vi "MaxiGauge EPICS2.vi"() -> ()   [LabVIEW 2015]
uses:
  <vilib>/Platform/TimedLoop/XDataNode/timing_clust.ctl
  <vilib>/Platform/TimedLoop/XDataNode/nitl_modes.ctl
  <vilib>/Platform/TimedLoop/XDataNode/wakeup.ctl
  <userlib>/caLab/Private/Get_PV-1D.vi
  <userlib>/caLab/Private/Put_DBL-1D_PV-1D.vi
  <vilib>/platform/TimedLoop/XDataNode/XDataNode.xnode
  <vilib>/Platform/TimedLoop/XDataNode/XDNodeRunTimeDep.lvlib
panel:
  out "Relay E":string
  out "Error out":errorcluster
  out "Maxigauge COMPORT":string
  out "APX:SEN6_STS":bool
  out "APX:SEN5_STS":bool
  out "APX:SEN4_STS":bool
  out "APX:SEN3_STS":bool
  out "APX:SEN2_STS":bool
  out "APX:SEN1_STS":bool
  out "APX:SEN6_VAL":dbl
  out "APX:SEN5_VAL":dbl
  out "APX:SEN4_VAL":dbl format="%#_3g"
  out "APX:SEN3_VAL":dbl format="%#_3g"
  out "APX:SEN2_VAL":dbl format="%#_3g"
  out "APX:SEN1_VAL":dbl
  out "APX:SEN6_OFF":bool
  out "APX:SEN6_ON":bool
  out "APX:SEN5_OFF":bool
  out "APX:SEN5_ON":bool
  out "APX:SEN4_OFF":bool
  out "APX:SEN4_ON":bool
  out "APX:SEN3_OFF":bool
  out "APX:SEN3_ON":bool
  out "APX:SEN2_OFF":bool
  out "APX:SEN2_ON":bool
  out "APX:SEN1_OFF":bool
  out "APX:SEN1_ON":bool
  out "APX:SP_SES100":bool
  out "MaxiGauge":dbl[](array[numeric])
  out "P torr":dbl[](array[numeric])
  in  "STOP":bool
  # "Ch 1\nGMP\nCh 6\nGMP\nCh 2\nGCC\nCh 4\nGHC\nCh 5\nGHC\n\nGMP"
  # "Send measured values to EPICS [COM8]"
  # "Relay E"
  # "K"
  # "EPICS PV name"
  # "N"
  # "APX:HPC100"
  # "APX:HPC100"
  # "APX:HPC01"
  # "APX:HPC"
  # "APX:HPC"
  # "N"
  # "APX:AP1"
  # "APX:PREP"
  # "APX:AP2"
  # "APX:Tsample"
  # "APX:AP1"
  # "APX:Tpiezo"
  # "APX:Thpc"
  # "APX:AP2"
  # "APX:PREP"
  # "APX:HPC01"
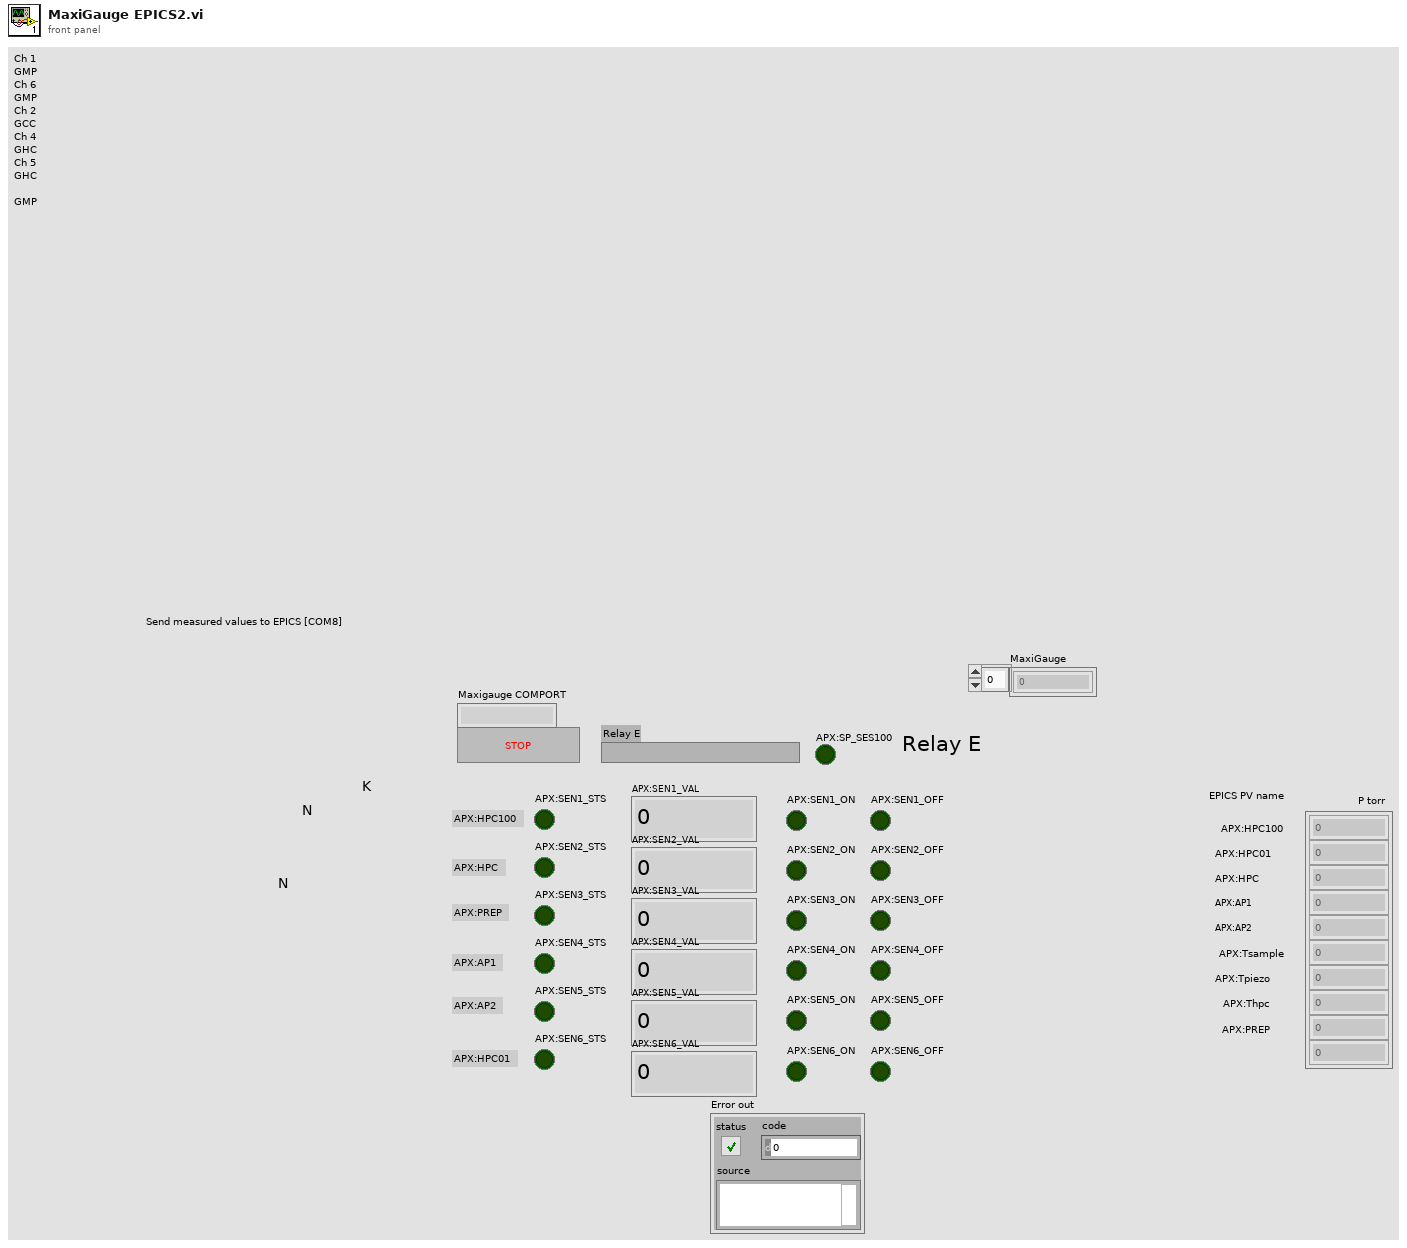
[diagram p1: front panel]
types:
  T1 = typedef "XDNodeRunTimeDep.lvlib/timing_clust.ctl" = cluster{"Expected End [f-1]":u64, "Actual End [f-1]":u64, "Finished Late? [f-1]":bool, "Expected End [i-1]":u64, "Actual End [i-1]":u64, "Finished Late? [i-1]":bool, "Expected Start [i]":u64, "Actual Start [i]":u64, "Expected Start [f]":u64, "Actual Start [f]":u64, "Source Name":string, "Structure Name":string, "Period":i64, "Deadline":i64, "Offset":i64, "Start":i64, "Priority":i32, "Timeout":i32, "Mode":T2, "Wakeup Reason":T3, "Error":errorcluster, "Source Type":string, "Secondary Source Type":string, "Global End Time":u64, "Global Start Time":u64, "Frame Duration":u64, "Iteration Duration":u64, "Assigned CPU":i32, "I/O Scan Engine Mode":u32}
  T2 = typedef "XDNodeRunTimeDep.lvlib/nitl_modes.ctl" = enum32{"No Change", "Process missed periods, maintain original phase", "Discard missed periods, maintain original phase", "Process missed periods, ignore original phase", "Discard missed periods, ignore original phase"}
  T3 = typedef "XDNodeRunTimeDep.lvlib/wakeup.ctl" = enum32{"Normal", "Aborted", "Asynchronous wakeup", "Timing source error", "Timed loop error", "Timeout"}
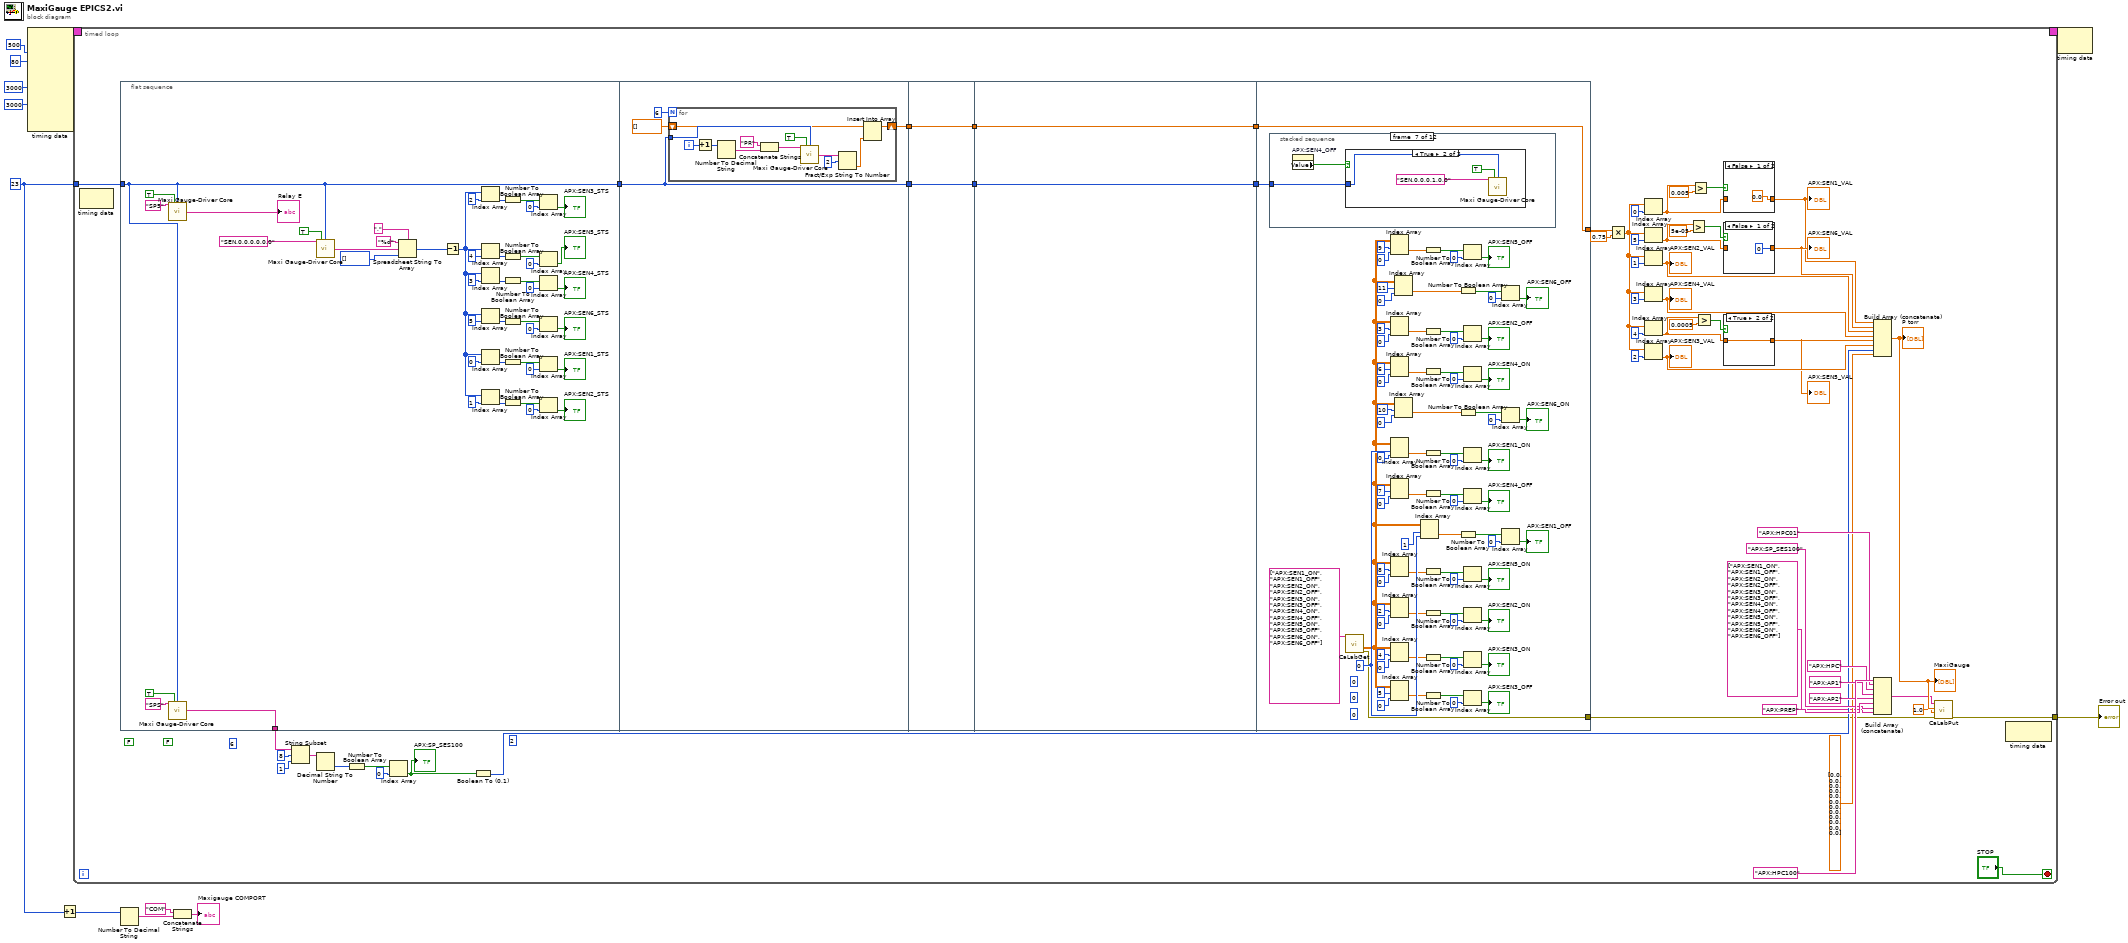
[diagram p0: block diagram]
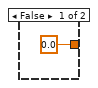
[diagram p2: hidden frame]
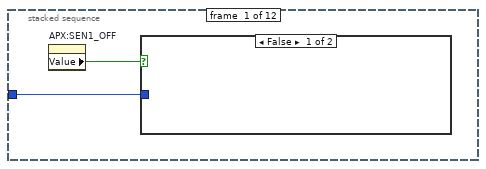
[diagram p3: hidden frame]
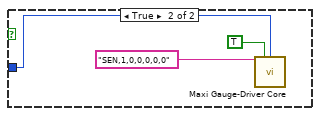
[diagram p4: hidden frame]
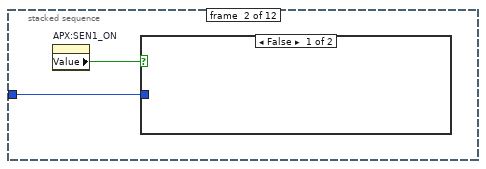
[diagram p5: hidden frame]
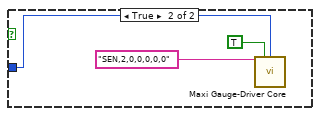
[diagram p6: hidden frame]
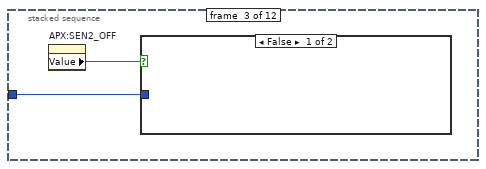
[diagram p7: hidden frame]
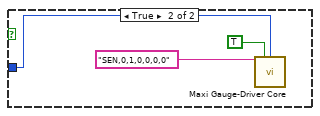
[diagram p8: hidden frame]
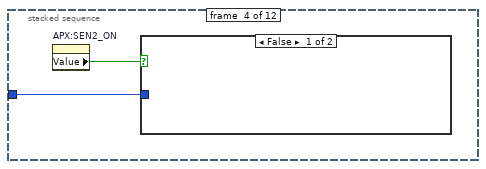
[diagram p9: hidden frame]
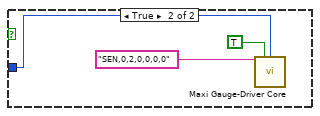
[diagram p10: hidden frame]
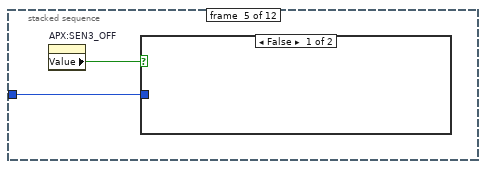
[diagram p11: hidden frame]
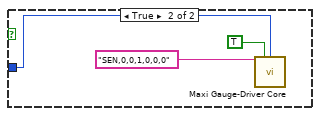
[diagram p12: hidden frame]
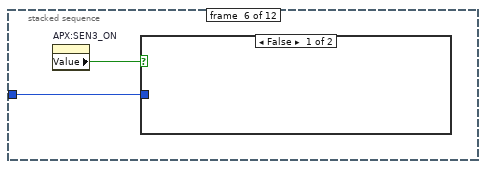
[diagram p13: hidden frame]
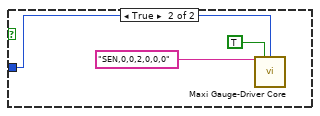
[diagram p14: hidden frame]
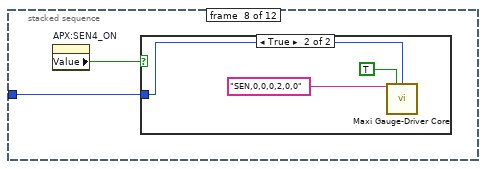
[diagram p16: hidden frame]
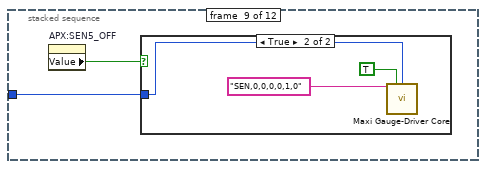
[diagram p18: hidden frame]
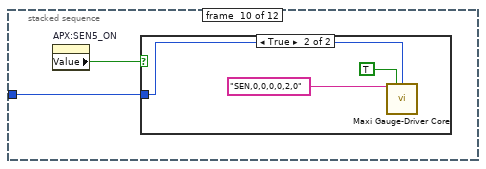
[diagram p20: hidden frame]
diagram:
  w8 = 23 ("Port")
  n1 = node-c288(i64 500 ("Period"), 80 ("Priority"), i64 3000 ("Deadline"), 3000 ("Timeout")) -> (w12:T1)  [unwired: 6 in]
  n2 = Increment(x=w8) -> (x+1=w7:i32)
  n3 = timed-loop {
    tunnel: w8 -> [w46]
    timing: w12 -> [_]
    timing-out: [_] -> w11
    tunnel: [w17] -> w3
    stop <- "STOP" stop-if-true
    (unwired) FALSE ("SES-100HVoff")
    (unwired) FALSE ("SES-100HVon")
    (unwired) 6
    (unwired) 2 ("index")
    n4 = node-c288() -> ()  [unwired: 1 in, 1 out]
    n5 = flat-sequence {
      tunnel: w46 -> [w73]
      tunnel: [w73] -> w45
      tunnel: [w113] -> w42
      tunnel: w45 -> [w116]
      tunnel: [w117] -> w22
      tunnel: [w116] -> w21
      tunnel: w22 -> [w133]
      tunnel: [w133] -> w16
      tunnel: w21 -> [w132]
      tunnel: [w132] -> w14
      tunnel: w16 -> [w135]
      tunnel: [w135] -> w15
      tunnel: w14 -> [w134]
      tunnel: [w134] -> w13
      tunnel: [w211] -> w58
      tunnel: w15 -> [w211]
      tunnel: w13 -> [w209]
      tunnel: [w136] -> w18
      frame #0 {
        n6 = call "Maxi Gauge-Driver Core.vi"("Command"="SP5", "Write/Read"=TRUE, "Port"=w73) -> ("String Out"=→"Relay E":string)  [unwired: 3 in, 9 out]
        n7 = call "Maxi Gauge-Driver Core.vi"("Command"="SPS", "Write/Read"=TRUE, "Port"=w73) -> ("String Out"=w113:string)  [unwired: 3 in, 9 out]
        n8 = call "Maxi Gauge-Driver Core.vi"("Command"="SEN,0,0,0,0,0,0", "Write/Read"=TRUE, "Port"=w73) -> ("String Out"=w109:string)  [unwired: 3 in, 9 out]
        n9 = Spreadsheet String To Array(delimiter (Tab)=",", format string="%d", spreadsheet string=w109, array type (2D Dbl)=i16[] []) -> (array=w105:i16[])
        n10 = Decrement(x=w105) -> (x-1=w80:i16[])
        n11 = Index Array(array=w80, index=2) -> (element=w95:i16)
        n12 = Index Array(array=w80, index=4) -> (element=w87:i16)
        n13 = Index Array(array=w80, index=3) -> (element=w91:i16)
        n14 = Index Array(array=w80, index=5) -> (element=w83:i16)
        n15 = Index Array(array=w80, index=0) -> (element=w104:i16)
        n16 = Index Array(array=w80, index=1) -> (element=w99:i16)
        n17 = Number To Boolean Array(number=w95) -> (Boolean array=w94:bool[])
        n18 = Number To Boolean Array(number=w87) -> (Boolean array=w86:bool[])
        n19 = Number To Boolean Array(number=w91) -> (Boolean array=w90:bool[])
        n20 = Number To Boolean Array(number=w83) -> (Boolean array=w82:bool[])
        n21 = Number To Boolean Array(number=w104) -> (Boolean array=w103:bool[])
        n22 = Number To Boolean Array(number=w99) -> (Boolean array=w98:bool[])
        n23 = Index Array(array=w94, index=0) -> (element=→"APX:SEN3_STS":bool)
        n24 = Index Array(array=w86, index=0) -> (element=→"APX:SEN5_STS":bool)
        n25 = Index Array(array=w90, index=0) -> (element=→"APX:SEN4_STS":bool)
        n26 = Index Array(array=w82, index=0) -> (element=→"APX:SEN6_STS":bool)
        n27 = Index Array(array=w103, index=0) -> (element=→"APX:SEN1_STS":bool)
        n28 = Index Array(array=w98, index=0) -> (element=→"APX:SEN2_STS":bool)
      }
      frame #1 {
        n29 = for {
          N: 6 -> [_]
          tunnel: w116 -> [w123]
          shift-right: [w120] -> w117
          shift-left: dbl[] [] -> [w121]
          i -> [w125]
          n30 = Increment(x=w125) -> (x+1=w128:i32)
          n31 = Number To Decimal String(number=w128) -> (decimal integer string=w131:string)  [unwired: 1 out]
          n32 = Concatenate Strings("PR", w131) -> (w129:string)
          n33 = call "Maxi Gauge-Driver Core.vi"("Command"=w129, "Write/Read"=TRUE, "Port"=w123) -> ("String Out"=w127:string)  [unwired: 3 in, 9 out]
          n34 = Fract/Exp String To Number(string=w127, offset=2 ("offset (0)")) -> (number=w122:dbl)  [unwired: 3 out]
          n35 = Insert Into Array(array=w121, new element=w122) -> (w120:dbl[])  [unwired: 1 in]
        }
      }
      frame #2 {
      }
      frame #3 {
      }
      frame #4 {
        (unwired) 0 ("index (col)")
        w199 = 0 ("index")
        (unwired) 0 ("disabled index (col)")
        (unwired) 0 ("index (row)")
        n36 = stacked-sequence {
          tunnel: w209 -> [w212 w217 w222 w227 w232 w237 w242 w247 w252 w257 w262 w267]
          frame #0 {
            n37 = property on="APX:SEN1_OFF" class="Bool (strict)"() -> ("Value"=w213:bool)  [unwired: 2 in, 2 out]
            n38 = case shown="False" w213 {
              tunnel: w212 -> [_ w214]
              frame False {
              }
              frame True {
                n39 = call "Maxi Gauge-Driver Core.vi"("Command"="SEN,1,0,0,0,0,0", "Write/Read"=TRUE, "Port"=w214) -> ()  [unwired: 3 in, 10 out]
              }
            }
          }
          frame #1 {
            n40 = property on="APX:SEN1_ON" class="Bool (strict)"() -> ("Value"=w218:bool)  [unwired: 2 in, 2 out]
            n41 = case shown="False" w218 {
              tunnel: w217 -> [_ w219]
              frame False {
              }
              frame True {
                n42 = call "Maxi Gauge-Driver Core.vi"("Command"="SEN,2,0,0,0,0,0", "Write/Read"=TRUE, "Port"=w219) -> ()  [unwired: 3 in, 10 out]
              }
            }
          }
          frame #2 {
            n43 = property on="APX:SEN2_OFF" class="Bool (strict)"() -> ("Value"=w223:bool)  [unwired: 2 in, 2 out]
            n44 = case shown="False" w223 {
              tunnel: w222 -> [_ w225]
              frame False {
              }
              frame True {
                n45 = call "Maxi Gauge-Driver Core.vi"("Command"="SEN,0,1,0,0,0,0", "Write/Read"=TRUE, "Port"=w225) -> ()  [unwired: 3 in, 10 out]
              }
            }
          }
          frame #3 {
            n46 = property on="APX:SEN2_ON" class="Bool (strict)"() -> ("Value"=w228:bool)  [unwired: 2 in, 2 out]
            n47 = case shown="False" w228 {
              tunnel: w227 -> [_ w230]
              frame False {
              }
              frame True {
                n48 = call "Maxi Gauge-Driver Core.vi"("Command"="SEN,0,2,0,0,0,0", "Write/Read"=TRUE, "Port"=w230) -> ()  [unwired: 3 in, 10 out]
              }
            }
          }
          frame #4 {
            n49 = property on="APX:SEN3_OFF" class="Bool (strict)"() -> ("Value"=w233:bool)  [unwired: 2 in, 2 out]
            n50 = case shown="False" w233 {
              tunnel: w232 -> [_ w234]
              frame False {
              }
              frame True {
                n51 = call "Maxi Gauge-Driver Core.vi"("Command"="SEN,0,0,1,0,0,0", "Write/Read"=TRUE, "Port"=w234) -> ()  [unwired: 3 in, 10 out]
              }
            }
          }
          frame #5 {
            n52 = property on="APX:SEN3_ON" class="Bool (strict)"() -> ("Value"=w238:bool)  [unwired: 2 in, 2 out]
            n53 = case shown="False" w238 {
              tunnel: w237 -> [_ w240]
              frame False {
              }
              frame True {
                n54 = call "Maxi Gauge-Driver Core.vi"("Command"="SEN,0,0,2,0,0,0", "Write/Read"=TRUE, "Port"=w240) -> ()  [unwired: 3 in, 10 out]
              }
            }
          }
          frame #6 {
            n55 = property on="APX:SEN4_OFF" class="Bool (strict)"() -> ("Value"=w243:bool)  [unwired: 2 in, 2 out]
            n56 = case shown="True" w243 {
              tunnel: w242 -> [_ w245]
              frame False {
              }
              frame True {
                n57 = call "Maxi Gauge-Driver Core.vi"("Command"="SEN,0,0,0,1,0,0", "Write/Read"=TRUE, "Port"=w245) -> ()  [unwired: 3 in, 10 out]
              }
            }
          }
          frame #7 {
            n58 = property on="APX:SEN4_ON" class="Bool (strict)"() -> ("Value"=w248:bool)  [unwired: 2 in, 2 out]
            n59 = case shown="True" w248 {
              tunnel: w247 -> [_ w250]
              frame False {
              }
              frame True {
                n60 = call "Maxi Gauge-Driver Core.vi"("Command"="SEN,0,0,0,2,0,0", "Write/Read"=TRUE, "Port"=w250) -> ()  [unwired: 3 in, 10 out]
              }
            }
          }
          frame #8 {
            n61 = property on="APX:SEN5_OFF" class="Bool (strict)"() -> ("Value"=w253:bool)  [unwired: 2 in, 2 out]
            n62 = case shown="True" w253 {
              tunnel: w252 -> [_ w255]
              frame False {
              }
              frame True {
                n63 = call "Maxi Gauge-Driver Core.vi"("Command"="SEN,0,0,0,0,1,0", "Write/Read"=TRUE, "Port"=w255) -> ()  [unwired: 3 in, 10 out]
              }
            }
          }
          frame #9 {
            n64 = property on="APX:SEN5_ON" class="Bool (strict)"() -> ("Value"=w258:bool)  [unwired: 2 in, 2 out]
            n65 = case shown="True" w258 {
              tunnel: w257 -> [_ w260]
              frame False {
              }
              frame True {
                n66 = call "Maxi Gauge-Driver Core.vi"("Command"="SEN,0,0,0,0,2,0", "Write/Read"=TRUE, "Port"=w260) -> ()  [unwired: 3 in, 10 out]
              }
            }
          }
          frame #10 {
            n67 = property on="APX:SEN6_OFF" class="Bool (strict)"() -> ("Value"=w263:bool)  [unwired: 2 in, 2 out]
            n68 = case shown="True" w263 {
              tunnel: w262 -> [_ w265]
              frame False {
              }
              frame True {
                n69 = call "Maxi Gauge-Driver Core.vi"("Command"="SEN,0,0,0,0,0,1", "Write/Read"=TRUE, "Port"=w265) -> ()  [unwired: 3 in, 10 out]
              }
            }
          }
          frame #11 {
            n70 = property on="APX:SEN6_ON" class="Bool (strict)"() -> ("Value"=w268:bool)  [unwired: 2 in, 2 out]
            n71 = case shown="True" w268 {
              tunnel: w267 -> [_ w270]
              frame False {
              }
              frame True {
                n72 = call "Maxi Gauge-Driver Core.vi"("Command"="SEN,0,0,0,0,0,2", "Write/Read"=TRUE, "Port"=w270) -> ()  [unwired: 3 in, 10 out]
              }
            }
          }
        }
        n73 = call-poly "CaLabGet.vi"("PV Names"=string[] ["APX:SEN1_ON", "APX:SEN1_OFF", "APX:SEN2_ON", "APX:SEN2_OFF", "APX:SEN3_ON", "APX:SEN3_OFF", "APX:SEN4_ON", "APX:SEN4_OFF", "APX:SEN5_ON", "APX:SEN5_OFF", "APX:SEN6_ON", "APX:SEN6_OFF"]) -> ("Value Array (number)"=w158:dbl[][], "Error out"=w136:errorcluster)  [unwired: 8 in, 5 out]
        n74 = Index Array(array=w158, index (row)=9 ("disabled index (col)"), index (col)=0) -> (element=w141:dbl)
        n75 = Index Array(array=w158, index (row)=3 ("disabled index (col)"), index (col)=0) -> (element=w153:dbl)
        n76 = Index Array(array=w158, index (row)=6 ("disabled index (col)"), index (col)=0) -> (element=w147:dbl)
        n77 = Index Array(array=w158, index (row)=w199, index (col)=0 ("disabled index (col)")) -> (element=w207:dbl)
        n78 = Index Array(array=w158, index (row)=7 ("disabled index (col)"), index (col)=0) -> (element=w145:dbl)
        n79 = Index Array(array=w158, index (row)=8 ("disabled index (col)"), index (col)=0) -> (element=w143:dbl)
        n80 = Index Array(array=w158, index (row)=2 ("disabled index (col)"), index (col)=0) -> (element=w155:dbl)
        n81 = Index Array(array=w158, index (row)=4 ("disabled index (col)"), index (col)=0) -> (element=w151:dbl)
        n82 = Index Array(array=w158, index (row)=5 ("disabled index (col)"), index (col)=0) -> (element=w149:dbl)
        n83 = Index Array(array=w158, index (row)=11 ("disabled index (col)"), index (col)=0) -> (element=w137:dbl)
        n84 = Index Array(array=w158, index (row)=10 ("disabled index (col)"), index (col)=0) -> (element=w139:dbl)
        n85 = Index Array(array=w158, index (row)=1 ("disabled index (col)"), index (col)=w199) -> (element=w203:dbl)
        n86 = Number To Boolean Array(number=w141) -> (Boolean array=w169:bool[])
        n87 = Number To Boolean Array(number=w153) -> (Boolean array=w193:bool[])
        n88 = Number To Boolean Array(number=w147) -> (Boolean array=w181:bool[])
        n89 = Number To Boolean Array(number=w207) -> (Boolean array=w206:bool[])
        n90 = Number To Boolean Array(number=w145) -> (Boolean array=w177:bool[])
        n91 = Number To Boolean Array(number=w143) -> (Boolean array=w173:bool[])
        n92 = Number To Boolean Array(number=w155) -> (Boolean array=w197:bool[])
        n93 = Number To Boolean Array(number=w151) -> (Boolean array=w189:bool[])
        n94 = Number To Boolean Array(number=w149) -> (Boolean array=w185:bool[])
        n95 = Number To Boolean Array(number=w137) -> (Boolean array=w161:bool[])
        n96 = Number To Boolean Array(number=w139) -> (Boolean array=w165:bool[])
        n97 = Number To Boolean Array(number=w203) -> (Boolean array=w202:bool[])
        n98 = Index Array(array=w169, index=0) -> (element=→"APX:SEN5_OFF":bool)
        n99 = Index Array(array=w193, index=0) -> (element=→"APX:SEN2_OFF":bool)
        n100 = Index Array(array=w181, index=0) -> (element=→"APX:SEN4_ON":bool)
        n101 = Index Array(array=w206, index=0) -> (element=→"APX:SEN1_ON":bool)
        n102 = Index Array(array=w177, index=0) -> (element=→"APX:SEN4_OFF":bool)
        n103 = Index Array(array=w173, index=0) -> (element=→"APX:SEN5_ON":bool)
        n104 = Index Array(array=w197, index=0) -> (element=→"APX:SEN2_ON":bool)
        n105 = Index Array(array=w189, index=0) -> (element=→"APX:SEN3_ON":bool)
        n106 = Index Array(array=w185, index=0) -> (element=→"APX:SEN3_OFF":bool)
        n107 = Index Array(array=w161, index=0) -> (element=→"APX:SEN6_OFF":bool)
        n108 = Index Array(array=w165, index=0) -> (element=→"APX:SEN6_ON":bool)
        n109 = Index Array(array=w202, index=0) -> (element=→"APX:SEN1_OFF":bool)
      }
    }
    n110 = String Subset(string=w42, offset (0)=8, length (rest)=1 ("length (rest)")) -> (substring=w38:string)
    n111 = Decimal String To Number(string=w38) -> (number=w39:i32)  [unwired: 2 in, 1 out]
    n112 = Number To Boolean Array(number=w39) -> (Boolean array=w41:bool[])
    n113 = Index Array(array=w41, index=0) -> (element=w37:bool)
    "APX:SP_SES100" <- w37
    n114 = Boolean To (0,1)(Boolean=w37) -> (0, 1=w28:i16)
    n115 = Multiply(x=w58, y=0.75) -> (x*y=w48:dbl[])
    n116 = Index Array(array=w48, index=0) -> (element=w36:dbl)
    n117 = Index Array(array=w48, index=5) -> (element=w33:dbl)
    n118 = Index Array(array=w48, index=1) -> (element=w35:dbl)
    "APX:SEN2_VAL" <- w35
    n119 = Index Array(array=w48, index=3) -> (element=w34:dbl)
    "APX:SEN4_VAL" <- w34
    n120 = Index Array(array=w48, index=4) -> (element=w26:dbl)
    n121 = Index Array(array=w48, index=2) -> (element=w30:dbl)
    "APX:SEN3_VAL" <- w30
    n122 = Greater?(x=w33, y=5e-05) -> (0:w62:bool)
    n123 = Greater?(x=w36, y=0.005) -> (0:w59:bool)
    n124 = Greater?(x=w26, y=0.0005) -> (0:w27:bool)
    n125 = case shown="False" w59 {
      tunnel: [0.0 w273] -> w23
      tunnel: w36 -> [_ w273]
      frame False {
      }
      frame True {
      }
    }
    "APX:SEN1_VAL" <- w23
    n126 = case shown="False" w62 {
      tunnel: [0 w275] -> w24
      tunnel: w33 -> [_ w275]
      frame False {
      }
      frame True {
      }
    }
    "APX:SEN6_VAL" <- w24
    n127 = case shown="True" w27 {
      tunnel: [0.0 w70] -> w25
      tunnel: w26 -> [_ w70]
      frame False {
      }
      frame True {
      }
    }
    "APX:SEN5_VAL" <- w25
    n128 = Build Array (concatenate)("APX:HPC100", "APX:HPC01", "APX:HPC", "APX:AP1", "APX:AP2", "APX:PREP", "APX:SP_SES100" ("element"), string[] ["APX:SEN1_ON", "APX:SEN1_OFF", "APX:SEN2_ON", "APX:SEN2_OFF", "APX:SEN3_ON", "APX:SEN3_OFF", "APX:SEN4_ON", "APX:SEN4_OFF", "APX:SEN5_ON", "APX:SEN5_OFF", "APX:SEN6_ON", "APX:SEN6_OFF"]) -> (w55:string[])
    n129 = Build Array (concatenate)(w23, w24, w35, w34, w25, w30, w28, dbl[] [0.0, 0.0, 0.0, 0.0, 0.0, 0.0, 0.0, 0.0, 0.0, 0.0, 0.0, 0.0]) -> (w56:dbl[])
    "P torr" <- w56
    "MaxiGauge" <- w56
    n130 = call-poly <userlib>:"CaLabPut.vi"("Error in (no error)"=w18, "Timeout (3)"=1.0, "Values"=w56, "PV Names"=w55) -> ("Error out"=w17:errorcluster)  [unwired: 4 in, 3 out]
    n131 = node-c288() -> ()  [unwired: 1 in, 1 out]
  }
  "Error out" <- w3
  n132 = Number To Decimal String(number=w7) -> (decimal integer string=w6:string)  [unwired: 1 in]
  n133 = Concatenate Strings("COM" ("string"), w6) -> (→"Maxigauge COMPORT":string)
  n134 = node-c288(w11) -> ()  [unwired: 1 out]
